vi "find vars in XML.vi"(10 "XML":string) -> (2 "Variables array":T1[](array[typedef]))   [LabVIEW 2015, in "Domino LM.lvlib" / "Domino Laser module Class.lvclass"]
uses:
  CTRLS/Domino Laser module Class.lvclass
  local printing/variable cluster.ctl
  CTRLS/GLB_VAR.vi
panel:
  out "Array":string[](array[string])
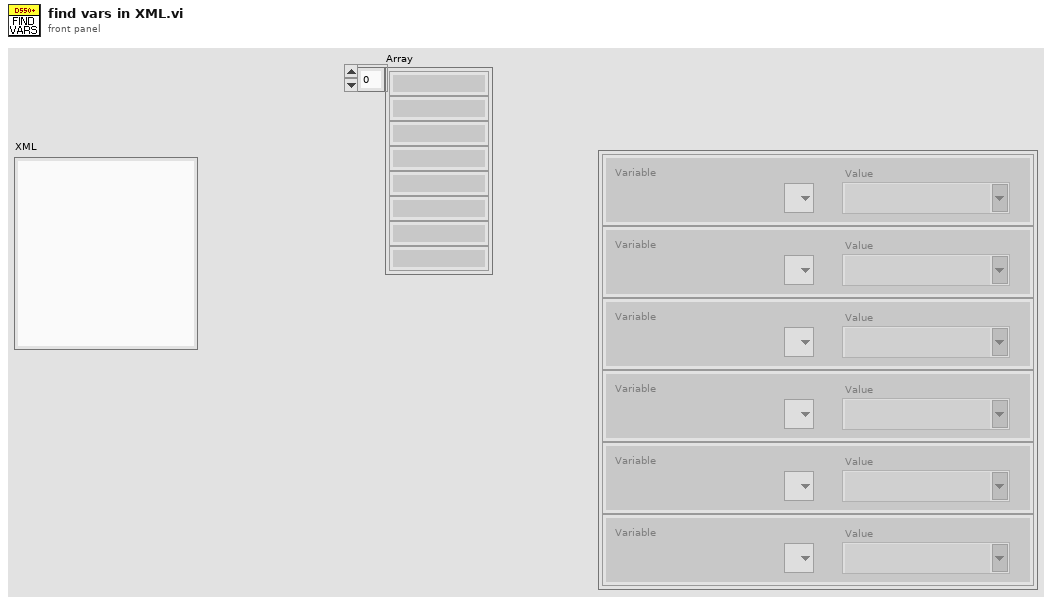
[diagram p1: front panel]
types:
  T1 = typedef "variable cluster.ctl" = cluster{"Variable":string, "Value":string}
  T2 = cluster{"User":cluster{"Username":refnum<vi>, "Password":refnum<vi>, "Current user":refnum<vi>, "user level":refnum<vi>, "Error MSG":refnum<vi>}, "Main":cluster{"Main Image":refnum<vi>, "Final Carton Status":refnum<vi>, "DM Status":refnum<vi>, "Serial Status":refnum<vi>, "Reject Reason":refnum<vi>, "Total Results":refnum<vi>, "Last Start Results":refnum<vi>, "DM Contents":refnum<vi>, "Motor Speed":refnum<vi>, "Batch Data":refnum<vi>, "Motor Status":refnum<vi>, "Stop Batch":refnum<vi>, "Start Batch":refnum<vi>, "Tab Control":refnum<vi>, "Check USB License":refnum<vi>, "OCV Status":refnum<vi>, "Printing Mode":refnum<vi>, "Variables array":refnum<vi>}, "Recipe":cluster{"Recipe_Carton":refnum<vi>, "Recipe_Printer":refnum<vi>, "Recipe_camera":refnum<vi>, "DM Elements":refnum<vi>, "IMG Config":refnum<vi>, "carton apply sucess":refnum<vi>, "Printer apply sucess":refnum<vi>, "Camera apply sucess":refnum<vi>, "DM Grade":refnum<vi>, "Line Elements":refnum<vi>, "Recipe Configuration":refnum<vi>, "Recipe Data":refnum<vi>, "Idle Button Enable":refnum<vi>, "Carton Config":refnum<vi>, "OCV Selection":refnum<vi>, "Layout Config":refnum<vi>, "Config local printing":refnum<vi>}, "Debug":cluster{"RT setpoints sucess":refnum<vi>, "speed mapping success ":refnum<vi>, "DM Search Options":refnum<vi>, "Speed Mapping":refnum<vi>, "Alarm Override":refnum<vi>, "Main Conv Speed":refnum<vi>, "PLC Settings":refnum<vi>, "Controller Setpoints":refnum<vi>, "Gate Location":refnum<vi>, "Image  Counter":refnum<vi>, "Signature  Counter":refnum<vi>, "Carton Width PLC [MM]":refnum<vi>, "Controller Inputs":refnum<vi>, "Controller Outputs":refnum<vi>}, "System":cluster{"Printer":refnum<vi>, "Printer apply sucess":refnum<vi>, "Camera apply sucess":refnum<vi>, "RT apply sucess":refnum<vi>, "Printer system sucess":refnum<vi>, "Camera Settings":refnum<vi>, "Camera system apply btn":refnum<vi>, "live img":refnum<vi>, "Scanner Settings":refnum<vi>, "Scanner apply sucess":refnum<vi>, "Scanner A Last MSG":refnum<vi>, "Scanner B Last MSG":refnum<vi>, "Emergency":refnum<vi>, "Shrould":refnum<vi>, "Printer Status":refnum<vi>, "OCV Select":refnum<vi>}, "Audit trail":cluster{"Audit filter cluster":refnum<vi>, "Audit Table":refnum<vi>}, "Batch":cluster{"New Workorder Data":refnum<vi>, "Edit Batch":refnum<vi>, "Close Batch":refnum<vi>, "Open Batch":refnum<vi>, "Create Batch":refnum<vi>, "SSCC Config":refnum<vi>}}
  T3 = cluster{"Work Order":string, "Recipe":string, "GTIN":string, "Batch":string, "Expiry Date":string, "MFG Date":string, "Case Count":string, "Sub Batch":string}
  T4 = cluster{"Layout File":string, "Date Separator":string, "Date Layout":string, "OCR Font":string, "Variable Data":string}
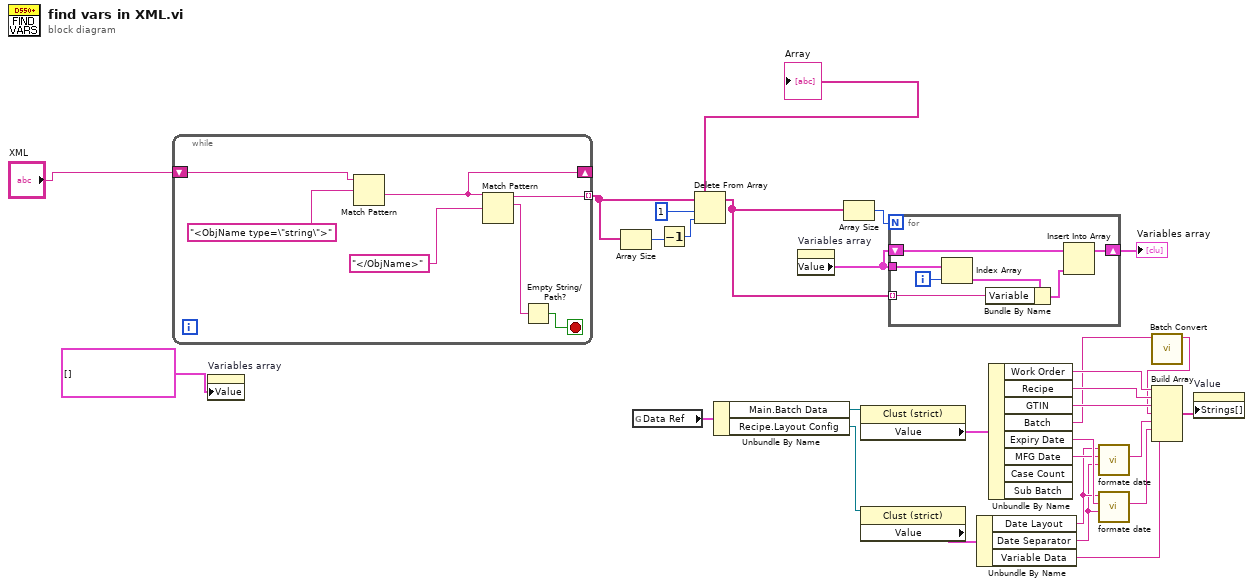
[diagram p0: block diagram]
diagram:
  n1 = while {
    tunnel: [w32] -> w26 mode=indexing
    shift-right: [w31] -> _
    shift-left: "XML" -> [w35]
    stop <- w29 stop-if-true
    n2 = Match Pattern(string=w35, regular expression="<ObjName type=\"string\">") -> (after substring=w31:string)  [unwired: 1 in, 3 out]
    n3 = Match Pattern(string=w31, regular expression="</ObjName>") -> (before substring=w32:string, match substring=w30:string)  [unwired: 1 in, 2 out]
    n4 = Empty String/Path?(string/path=w30) -> (empty?=w29:bool)
  }
  n5 = property on="Variables array" class="Arr (strict)"("Value"=T1[] [] ("Variables array")) -> ()  [unwired: 2 in, 2 out]
  n6 = Array Size(array=w26) -> (size(s)=w25:i32)
  n7 = global read "GLB_VAR.vi" "Data Ref"() -> (w18:T2)
  n8 = Decrement(x=w25) -> (x-1=w24:i32)
  n9 = Delete From Array(array=w26, length=1, index=w24) -> (array with subset deleted=w23:string[])  [unwired: 1 out]
  "Array" <- w23
  n10 = Unbundle By Name(w18) -> ("Main.Batch Data"=w17:refnum<vi>, "Recipe.Layout Config"=w15:refnum<vi>)
  n11 = property on="Variables array" class="Arr (strict)"() -> ("Value"=w21:T1[])  [unwired: 2 in, 2 out]
  n12 = Array Size(array=w23) -> (size(s)=w22:i32)
  n13 = property class="Clust (strict)"(reference=w17) -> ("Value"=w16:T3)  [unwired: 1 in, 2 out]
  n14 = property class="Clust (strict)"(reference=w15) -> ("Value"=w14:T4)  [unwired: 1 in, 2 out]
  n15 = for {
    N: w22 -> [_]
    tunnel: w21 -> [w38]
    tunnel: w23 -> [w42] mode=indexing
    shift-right: [w39] -> w20
    shift-left: w21 -> [w41]
    i -> [w37]
    n16 = Index Array(array=w38, index=w37) -> (element=w36:T1)
    n17 = Bundle By Name(cluster=w36, "Variable"=w42) -> (w40:T1)
    n18 = Insert Into Array(array=w41, new element=w40) -> (w39:T1[])  [unwired: 1 in]
  }
  "Variables array" <- w20
  n19 = Unbundle By Name(w14) -> ("Date Layout"=w11:string, "Date Separator"=w10:string, "Variable Data"=w3:string)
  n20 = Unbundle By Name(w16) -> ("Work Order"=w9:string, "Recipe"=w8:string, "GTIN"=w7:string, "Batch"=w2:string, "Expiry Date"=w13:string, "MFG Date"=w12:string)  [unwired: 2 out]
  n21 = call "formate date.vi"("Sepertaor"=w10, "Input Date"=w12, "Layout"=w11) -> ("Formatted Date"=w6:string)  [unwired: 8 in]
  n22 = call "formate date.vi"("Sepertaor"=w10, "Input Date"=w13, "Layout"=w11) -> ("Formatted Date"=w5:string)  [unwired: 8 in]
  n23 = call "Batch Convert.vi"("Batch"=w2) -> ("string"=w1:string)  [unwired: 10 in]
  n24 = Build Array(w9, w8, w7, w1, w6, w5, w3) -> (w4:string[])
  n25 = property on="Value" class="CmbBox"("Strings[]"=w4) -> ()  [unwired: 2 in, 2 out]
